vi "Accelerator DML Complex Process.vi"(9 "Sessions Parameters":T1={"intra_op_num_threads"=0, "inter_op_num_threads"=0, "execution_mode"=enum."ORT_SEQUENTIAL", "deterministic_compute"=FALSE, "graph_optimization_level"=1, "optimized_model_file_path"=path "", "profiling output dir"=path ""} {"graph_optimization_level" items=["ORT_DISABLE_ALL"=0, "ORT_ENABLE_ALL"=1, "ORT_ENABLE_BASIC"=2, "ORT_ENABLE_EXTENDED"=99]}, 11 "X size":i32=16384) -> (3 "Accelerator Time":dbl=0.19947869999998602)   [LabVIEW 2020]
uses:
  <vilib>/Graiphic/Accelerator/Source/SubVIs/add_to_cluster_onnx_input/acc_onnx_add_1d_complexfloat_array_into_input_cluster_array_by_idx.vi
  <vilib>/Graiphic/Accelerator/Source/Model/_Methods/acc_create_onnx_model_then_init_dml_inference_session.vi
  <vilib>/Graiphic/Accelerator/Source/SubVIs/add_to_cluster_onnx_input/acc_onnx_add_scalar_complexfloat_array_into_input_cluster_array_by_idx.vi
  <vilib>/Graiphic/Accelerator/Source/ONNX/Inference/_Methods/Simplified/acc_embedded_run_preallocated_multi_input_and_outputs_dml_by_idx.vi
  <vilib>/Graiphic/Accelerator/Source/ONNX/Inference/_Methods/Exec_DML/acc_embedded_copy_dml_ptr_data_to_labview_data.vi
  <vilib>/Graiphic/Accelerator/Source/ONNX/Inference/_Methods/Simplified/acc_embedded_run_mono_output_scalar_complexfloat.vi
  <vilib>/Graiphic/Accelerator/Source/ONNX/Inference/acc_Inference.lvclass
  <vilib>/Analysis/NI_AALBase.lvlib
  <vilib>/Graiphic/Accelerator/Source/Model/acc_Model.lvclass
panel:
  out "max value":csg=5.4420166+0.0i
  in  "nb_loop":i32=6
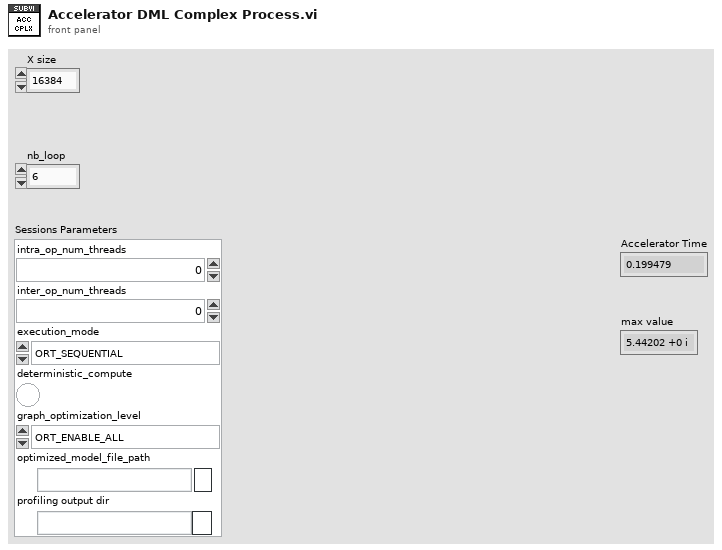
[diagram p1: front panel]
types:
  T1 = cluster{"intra_op_num_threads":i32, "inter_op_num_threads":i32, "execution_mode":enum16{"ORT_SEQUENTIAL", "ORT_PARALLEL"}, "deterministic_compute":bool, "graph_optimization_level":u16, "optimized_model_file_path":path, "profiling output dir":path}
  T2 = typedef "acc_onnx_multi_input_index_cluster.ctl" = cluster{"input_order":u32, "Inputs Info":cluster{"inputs_data":u8[], "inputs_shapes":i64[], "inputs string length":i64[], "inputs_ranks":i64[], "inputs_types":T3[]}}
  T3 = typedef "acc_onnx_dtype_enum.ctl" = enum16{"UNDEFINED", "FLOAT", "UINT8", "INT8", "UINT16", "INT16", "INT32", "INT64", "STRING", "BOOL", "FLOAT16", "DOUBLE", "UINT32", "UINT64", "COMPLEX64", "COMPLEX128", "BFLOAT16", "FLOAT8E4M3FN", "FLOAT8E4M3FNUZ", "FLOAT8E5M2", "FLOAT8E5M2FNUZ", "UINT4", "INT4"}
  T4 = typedef "acc_onnx_multi_ptr_input_index_cluster.ctl" = cluster{"input_order":u32, "Inputs Info":cluster{"inputs_ptr":u64, "inputs_shapes":i64[], "inputs_ranks":i64, "inputs_types":T3}}
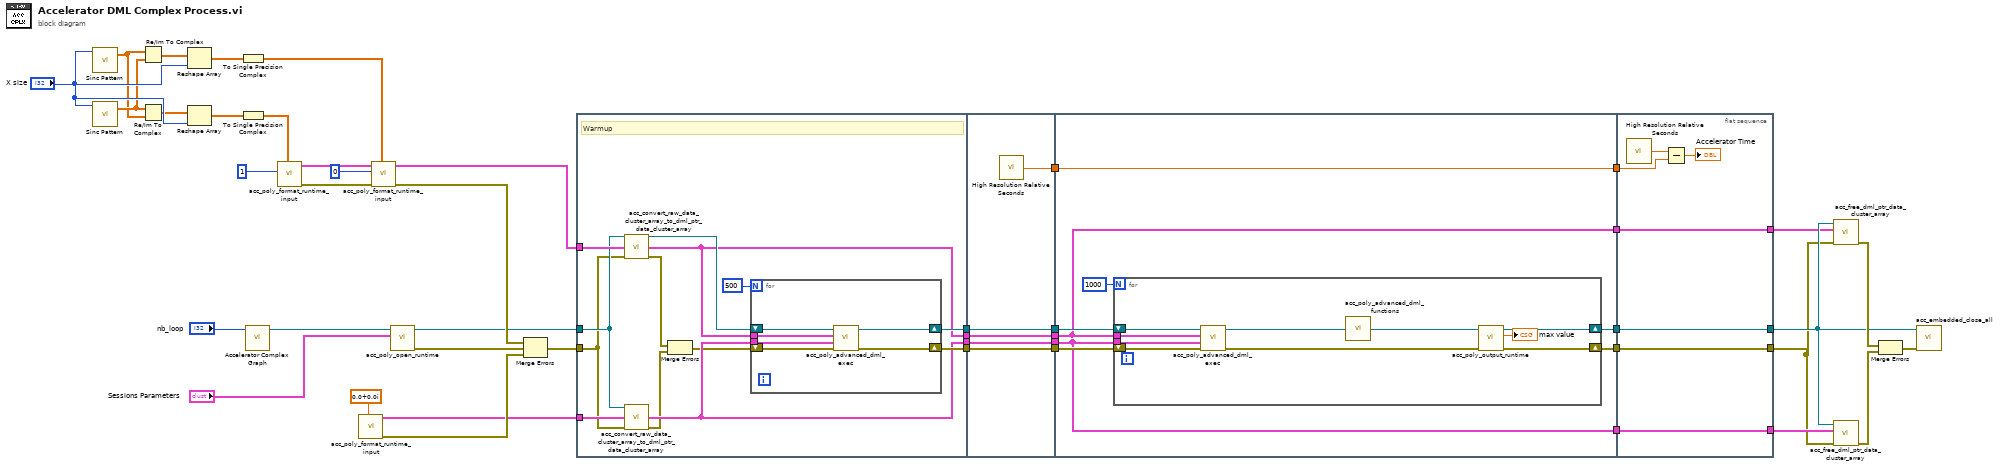
[diagram p0: block diagram]
diagram:
  n1 = call <vilib>:"Sinc Pattern.vi"("samples"="X size") -> ("Sinc Pattern"=w35:dbl[])  [unwired: 3 in, 1 out]
  n2 = call <vilib>:"Sinc Pattern.vi"("samples"="X size") -> ("Sinc Pattern"=w36:dbl[])  [unwired: 3 in, 1 out]
  n3 = Re/Im To Complex(1:w36, 2:w35) -> (0:w37:cdb[])
  n4 = Re/Im To Complex(1:w35, 2:w36) -> (0:w34:cdb[])
  n5 = Reshape Array(w37, "X size") -> (w33:cdb[])
  n6 = Reshape Array(w34, "X size") -> (w32:cdb[])
  n7 = To Single Precision Complex(1:w33) -> (0:w30:csg[])
  n8 = To Single Precision Complex(1:w32) -> (0:w31:csg[])
  n9 = call "Accelerator Complex Graph.vi"("nb_loop"="nb_loop") -> ("Model out"=w28:refnum<class "acc_Model.lvclass">)  [unwired: 10 in]
  n10 = call-poly <vilib>:"acc_poly_format_runtime_input.vi"("1D Input Data"=w31, "input order"=1) -> ("error out"=w42:errorcluster, "Data out (Fwd in)"=w43:T2[])  [unwired: 8 in]
  n11 = call-poly <vilib>:"acc_poly_format_runtime_input.vi"("Input Data"=csg 0.0+0.0i) -> ("error out"=w38:errorcluster, "Data out (Fwd in)"=w8:T2[])  [unwired: 9 in]
  n12 = call-poly <vilib>:"acc_poly_format_runtime_input.vi"("1D Input Data"=w30, "error in"=w42, "input order"=0, "Data in"=w43) -> ("error out"=w39:errorcluster, "Data out (Fwd in)"=w11:T2[])  [unwired: 6 in]
  n13 = call-poly <vilib>:"acc_poly_open_runtime.vi"("Sessions Parameters"="Sessions Parameters", "Model in"=w28) -> ("error out"=w27:errorcluster, "Inference out"=w9:refnum<class "acc_Inference.lvclass">)  [unwired: 8 in]
  n14 = Merge Errors(w39, w27, w38) -> (w10:errorcluster)
  n15 = flat-sequence {
    tunnel: w10 -> [w49]
    tunnel: w11 -> [w54]
    tunnel: w8 -> [w53]
    tunnel: w9 -> [w52]
    tunnel: [w58] -> w25
    tunnel: [w51] -> w24
    tunnel: [w57] -> w23
    tunnel: [w50] -> w22
    tunnel: [w69] -> w21
    tunnel: [w68] -> w20
    tunnel: [w67] -> w19
    tunnel: [w66] -> w18
    tunnel: [w65] -> w17
    tunnel: w25 -> [w68]
    tunnel: w24 -> [w67]
    tunnel: w23 -> [w65]
    tunnel: w22 -> [w66]
    tunnel: w21 -> [w77]
    tunnel: [w77] -> w16
    tunnel: w20 -> [w75]
    tunnel: w19 -> [w70]
    tunnel: w18 -> [w71]
    tunnel: w17 -> [w74]
    tunnel: [w73] -> w15
    tunnel: [w72] -> w14
    tunnel: [w71] -> w13
    tunnel: [w70] -> w12
    tunnel: w16 -> [w93]
    tunnel: [w91] -> w3
    tunnel: w15 -> [w91]
    tunnel: w14 -> [w90]
    tunnel: [w90] -> w2
    tunnel: [w89] -> w1
    tunnel: w13 -> [w89]
    tunnel: [w88] -> w4
    tunnel: w12 -> [w88]
    frame #0 {
      # "Warmup"
      n16 = call <vilib>:"acc_convert_raw_data_cluster_array_to_dml_ptr_data_cluster_array.vi"("Inference in"=w52, "Data in"=w54, "error in"=w49) -> ("Inference out"=w55:refnum<class "acc_Inference.lvclass">, "Data in"=w50:T4[], "error out"=w46:errorcluster)  [unwired: 10 in]
      n17 = call <vilib>:"acc_convert_raw_data_cluster_array_to_dml_ptr_data_cluster_array.vi"("Inference in"=w52, "Data in"=w53, "error in"=w49) -> ("Data in"=w51:T4[], "error out"=w48:errorcluster)  [unwired: 10 in, 1 out]
      n18 = Merge Errors(w46, w48) -> (w47:errorcluster)
      n19 = for {
        N: 500 -> [_]
        tunnel: w50 -> [w61]
        tunnel: w51 -> [w60]
        shift-right: [w63] -> w58
        shift-left: w55 -> [w64]
        shift-right: [w59] -> w57
        shift-left: w47 -> [w62]
        n20 = call-poly <vilib>:"acc_poly_advanced_dml_exec.vi"("error in"=w62, "Data out"=w60, "Data in"=w61, "Inference in"=w64) -> ("error out"=w59:errorcluster, "Inference out"=w63:refnum<class "acc_Inference.lvclass">)  [unwired: 6 in]
      }
    }
    frame #1 {
      n21 = call <vilib>:"High Resolution Relative Seconds.vi"() -> ("relative seconds"=w69:dbl)
    }
    frame #2 {
      n22 = for {
        N: 1000 -> [_]
        tunnel: w70 -> [w86]
        tunnel: w71 -> [w85]
        shift-right: [w81] -> w73
        shift-left: w75 -> [w87]
        shift-right: [w80] -> w72
        shift-left: w74 -> [w84]
        n23 = call-poly <vilib>:"acc_poly_advanced_dml_exec.vi"("error in"=w84, "Data out"=w86, "Data in"=w85, "Inference in"=w87) -> ("error out"=w82:errorcluster, "Inference out"=w83:refnum<class "acc_Inference.lvclass">)  [unwired: 6 in]
        n24 = call-poly <vilib>:"acc_poly_advanced_dml_functions.vi"("Inference in"=w83) -> ("Inference out"=w79:refnum<class "acc_Inference.lvclass">)
        n25 = call-poly <vilib>:"acc_poly_output_runtime.vi"("error in"=w82, "Inference in"=w79) -> ("error out"=w80:errorcluster, "Output Data"=→"max value":csg, "Inference out"=w81:refnum<class "acc_Inference.lvclass">)  [unwired: 7 in]
      }
    }
    frame #3 {
      n26 = call <vilib>:"High Resolution Relative Seconds.vi"() -> ("relative seconds"=w94:dbl)
      n27 = Subtract(x=w94, y=w93) -> (x-y=→"Accelerator Time":dbl)
    }
  }
  n28 = call <vilib>:"acc_free_dml_ptr_data_cluster_array.vi"("error in"=w2, "Data in"=w1, "Inference in"=w3) -> ("error out"=w6:errorcluster)  [unwired: 7 in, 1 out]
  n29 = call <vilib>:"acc_free_dml_ptr_data_cluster_array.vi"("error in"=w2, "Data in"=w4, "Inference in"=w3) -> ("error out"=w7:errorcluster)  [unwired: 7 in, 1 out]
  n30 = Merge Errors(w6, w7) -> (w5:errorcluster)
  n31 = call-dynamic "acc_embedded_close_all.vi"("error in"=w5, "Inference in"=w3) -> ()  [unwired: 8 in, 2 out]
